vi "init.vi"(8 "error in (no error)":errorcluster, 10 "Init Data":variant, 11 "Temp Control in":refnum<class "Temp Control.lvclass">) -> (0 "error out":errorcluster, 2 "Channel List":refnum<class "HK Item.lvclass">[](array[class]), 3 "Temp Control out":refnum<class "Temp Control.lvclass">)   [LabVIEW 2022 SP3, in "Temp Control.lvclass"]
uses:
  Temp Control.lvclass
  hk-channel-class/hk-channel-class/HK Item/HK Item.lvclass
  Temp Control.lvclass/Temp Control.ctl
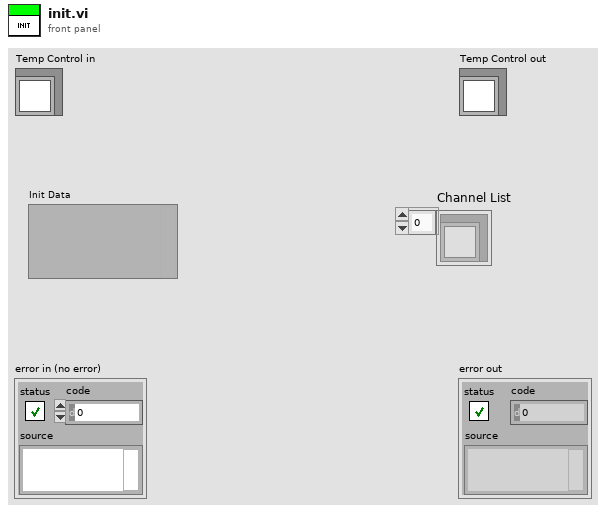
[diagram p1: front panel]
types:
  T1 = typedef "Temp Control.lvclass/Temp Control Sim Settings.ctl" = cluster{"Offsets out":dbl[], "Scaling out":dbl[]}
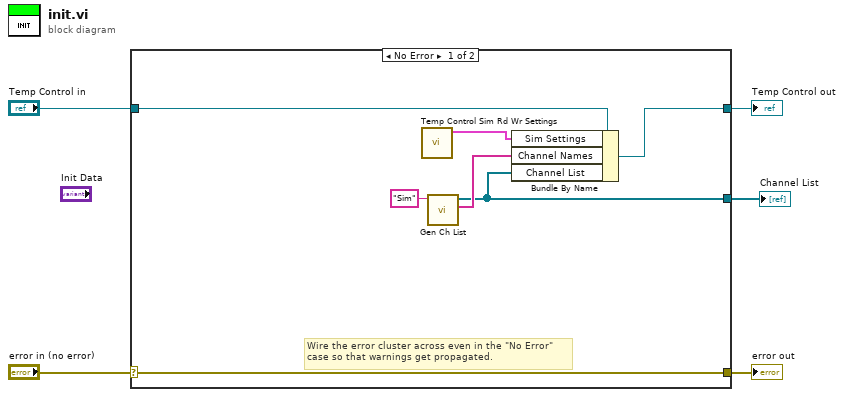
[diagram p0: block diagram]
diagram:
  n1 = case shown="No Error" "error in (no error)" {
    selector: "error in (no error)" -> [w12 w14]
    tunnel: [w12 w14] -> w4
    tunnel: [w9 w13] -> w2
    tunnel: "Temp Control in" -> [w8 w13]
    tunnel: [w10 _] -> w1
    frame No Error {
      # "Wire the error cluster across even in the \"No Error\"\ncase so that warnings get propagated."
      n2 = call "Temp Control Sim Rd Wr Settings.vi"() -> ("Sim Settings"=w6:T1)  [unwired: 10 in, 1 out]
      n3 = call "Gen Ch List.vi"("Prefix"="Sim") -> ("Channel Names"=w11:string[], "Channel List"=w10:refnum<class "HK Item.lvclass">[])  [unwired: 9 in]
      n4 = Bundle By Name(cluster=w8, "Sim Settings"=w6, "Channel Names"=w11, "Channel List"=w10) -> (w9:refnum<class "Temp Control.lvclass">)
    }
    frame Error {
    }
  }
  "error out" <- w4
  "Temp Control out" <- w2
  "Channel List" <- w1
